vi "Solve General Complex Linear Equations By LU.vi"(3 "Known Vector":cdb[](array[numeric]) format="%.2f", 4 "Input Matrix":T1) -> (0 "error":i32, 1 "Solution Vector":cdb[](array[numeric]) format="%.2f")   [LabVIEW 2017, in "NI_AALBase.lvlib"]
doc: "Solves a complex linear system AX=Y using LU factorization."
uses:
  NI_AALBase.lvlib
  ComplexMatrix.ctl
  <resource>/lvanlys.dll
  NI_Matrix.lvlib
panel:
  # "Solve General Complex Linear Equations"
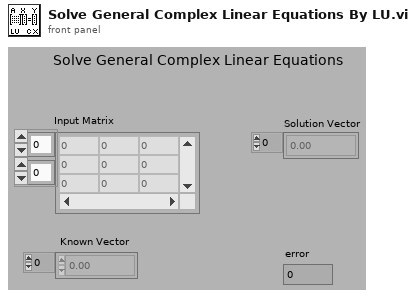
[diagram p1: front panel]
types:
  T1 = typedef "NI_Matrix.lvlib/ComplexMatrix.ctl" = cdb[][]
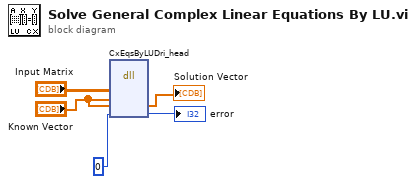
[diagram p0: block diagram]
diagram:
  n1 = dll-call lib="C:/Program Files (x86)/National Instruments/LabVIEW 2017/resource/lvanlys.*" fn="CxEqsByLUDri_head"("Input Matrix"="Input Matrix", "Known Vector"="Known Vector", "Known Vector"="Known Vector", 0) -> ("Known Vector"=→"Solution Vector":cdb[], →"error":i32)  [unwired: 6 in, 2 out]
